vi "Main.vi"(11 "DataIn":T1) -> (3 "DataOut":T1)   [LabVIEW 2018]
doc: "Main Vi para Jogo da Velha Multiplayer - Player x Player na mesma máquina, Player x Player pela rede, Player x Computador\n[Covers: REQ05]"
uses:
  controls/Tabuleiro.ctl
  controls/DataIn.ctl
  MatchDataClasses/MatchData/MatchData.lvclass
  controls/GameOption.ctl
  controls/Table.ctl
  controls/States.ctl
  controls/LogStates.ctl
  MatchDataClasses/Local/Local.lvclass
  C:/Users/liferrei/Documents/Jogo-da-Velha/MatchDataClasses/MatchData/MatchData.lvclass
  MatchDataClasses/Remote/Remote.lvclass
  Globals.vi
panel:
  in  "Remote?":bool
  in  "Reiniciar":bool
  out "Quem joga":string
  out "Tabuleiro":T2
  # "JOGO DA VELHA"
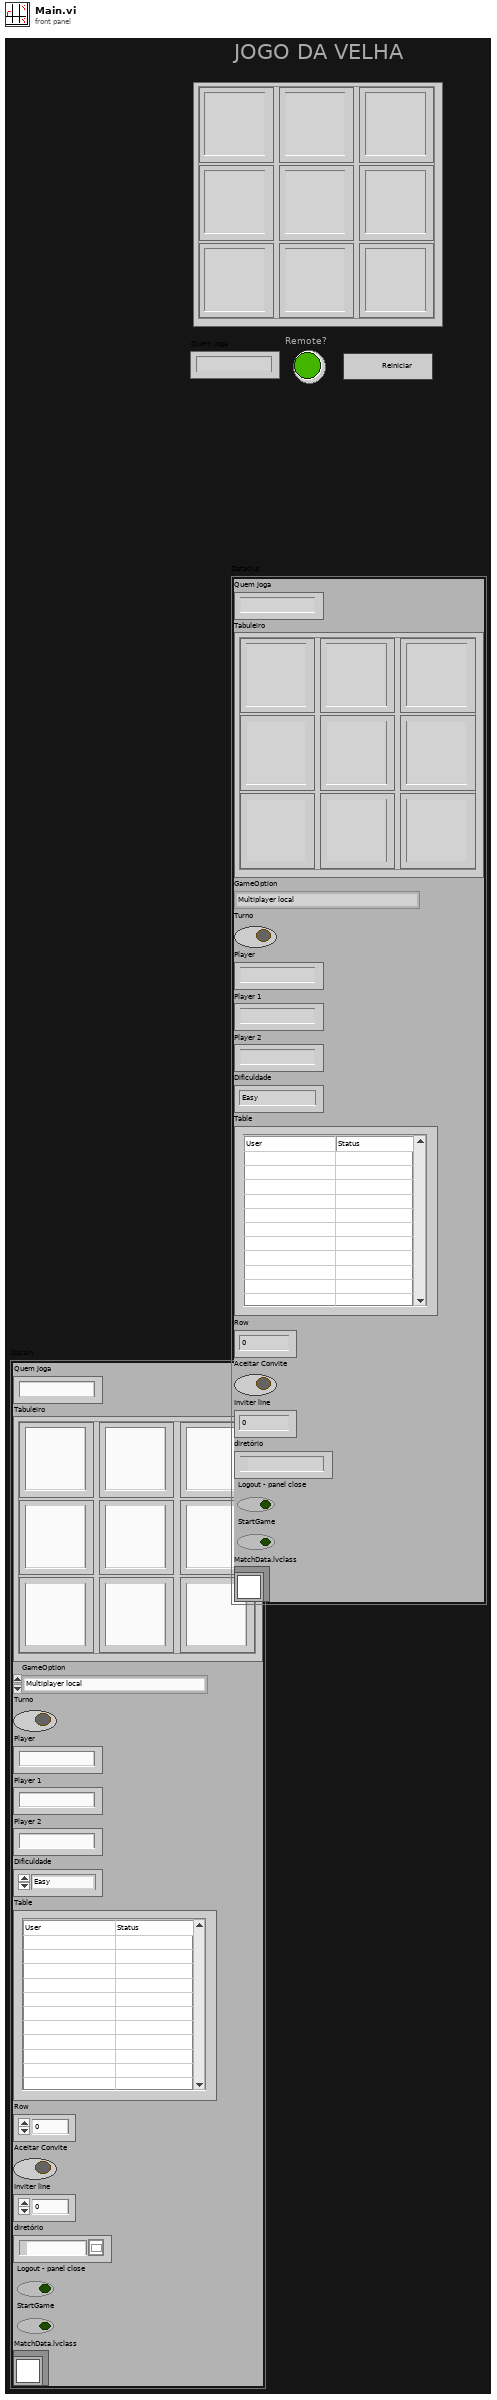
[diagram p1: front panel]
types:
  T1 = typedef "DataIn.ctl" = cluster{"Quem Joga":string, "Tabuleiro":T2, "GameOption":T3, "Turno":bool, "Player":string, "Player 1":string, "Player 2":string, "Dificuldade":enum16{"Easy", "Medium", "Hard"}, "Table":T4, "Row":u32, "Aceitar Convite":bool, "Inviter line":u32, "diretório":path, "Logout - panel close":bool, "StartGame":bool, "MatchData.lvclass":refnum<class "MatchData.lvclass">}
  T2 = typedef "Tabuleiro.ctl" = cluster{"(0,0)":string, "(1,0)":string, "(0,1)":string, "(1,1)":string, "(2,0)":string, "(1,2)":string, "(2,2)":string, "(0,2)":string, "(2,1) ":string}
  T3 = typedef "GameOption.ctl" = enum16{"Multiplayer local", "Multiplayer remoto", "Single Player", "Wait for Event", "Initialize", "Stop"}
  T4 = typedef "Table.ctl" = string[][]
  T5 = typedef "States.ctl" = enum16{"Initialize", "Player (wait for event)", "Stop", "PC", "Restart"}
  T6 = typedef "LogStates.ctl" = enum16{"Initialize", "Write", "Write (win, draw)", "Write (PC first)", "Write (Player first)", "Close"}
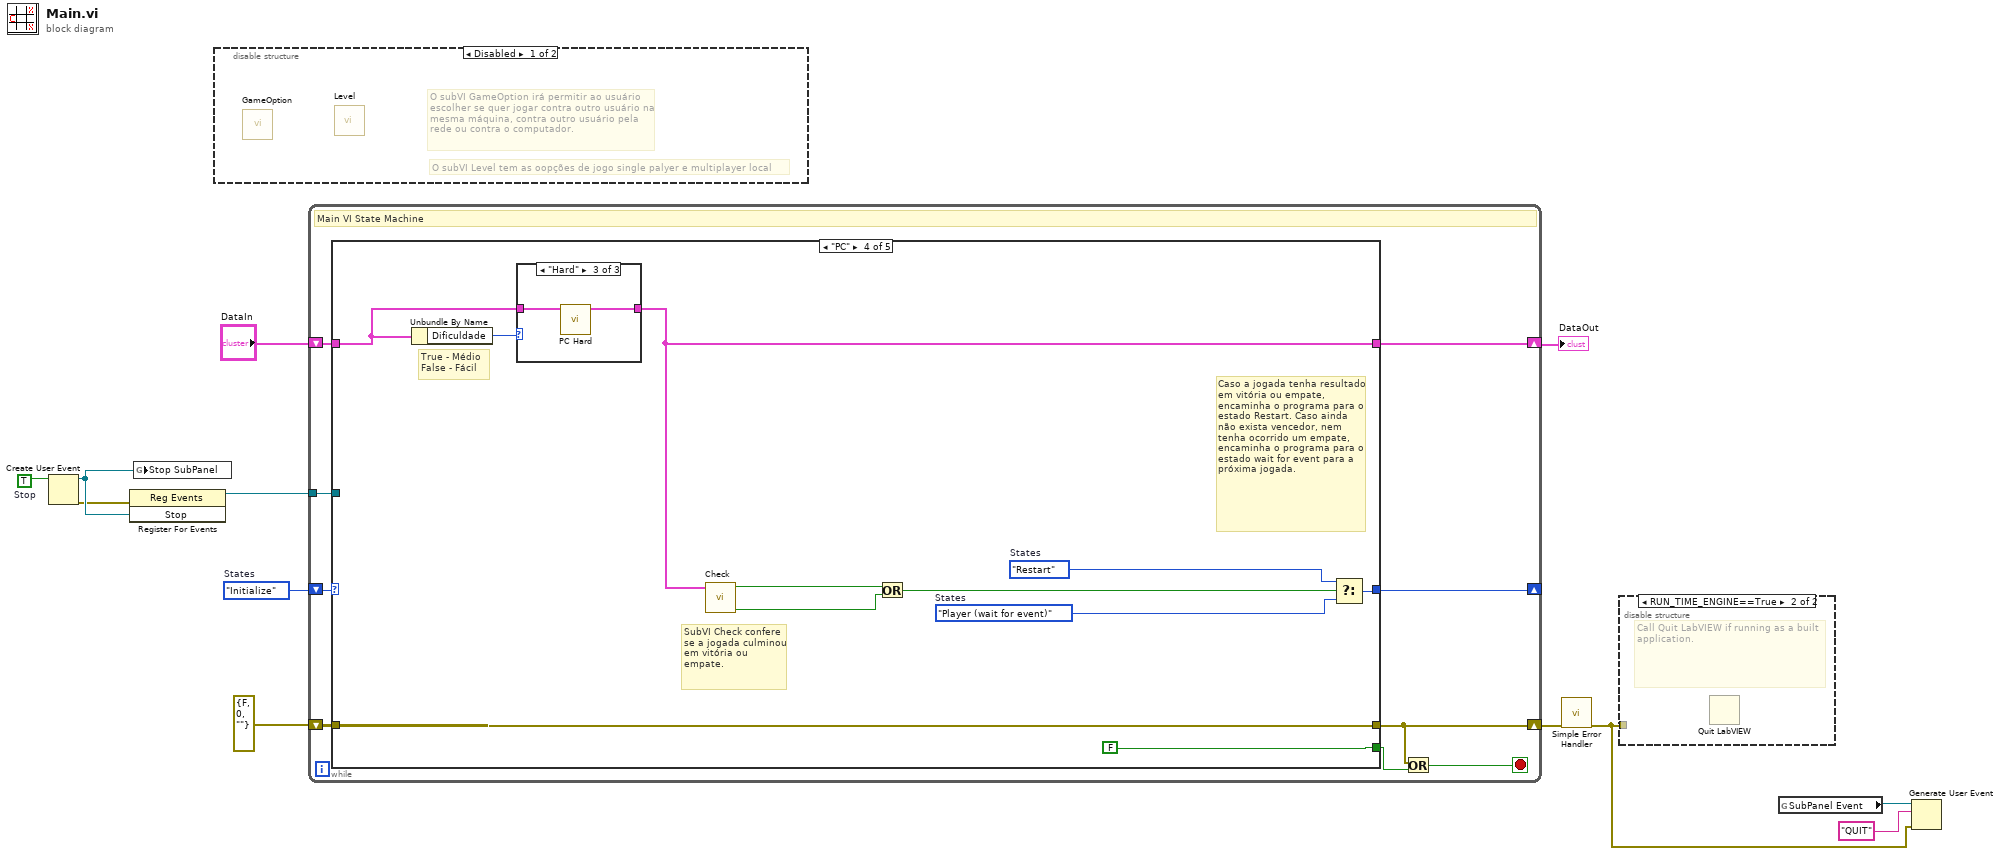
[diagram p0: block diagram]
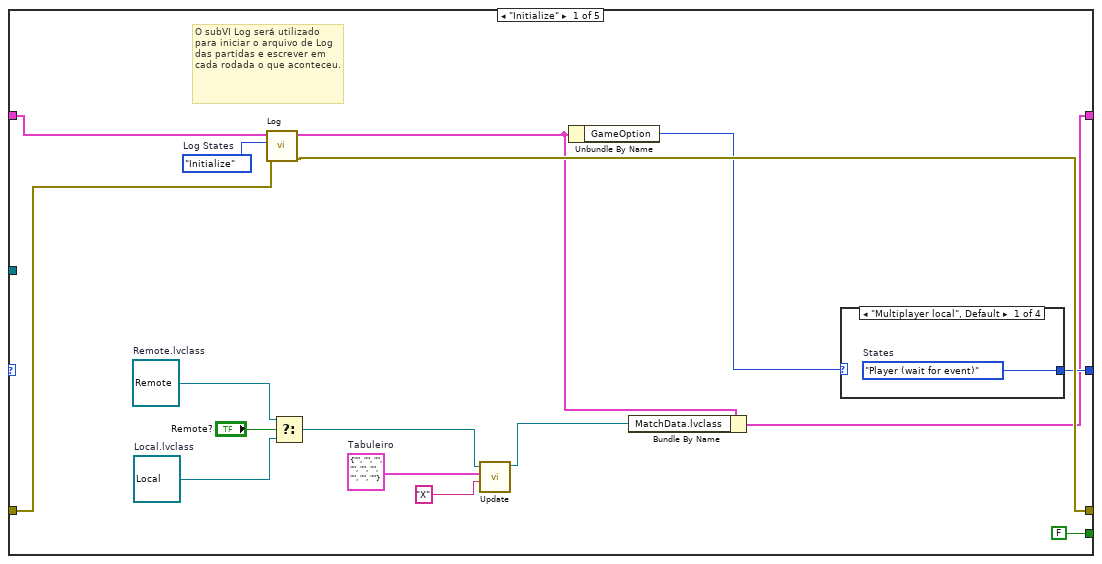
[diagram p3: hidden frame]
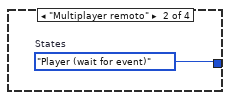
[diagram p4: hidden frame]
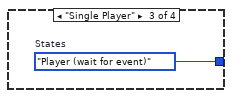
[diagram p5: hidden frame]
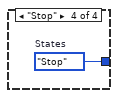
[diagram p6: hidden frame]
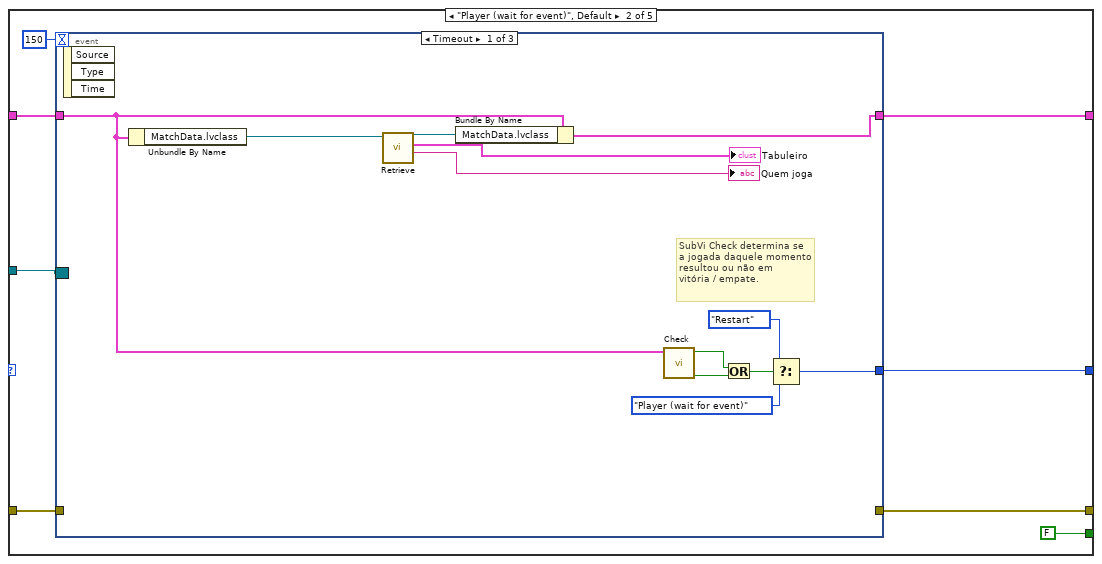
[diagram p7: hidden frame]
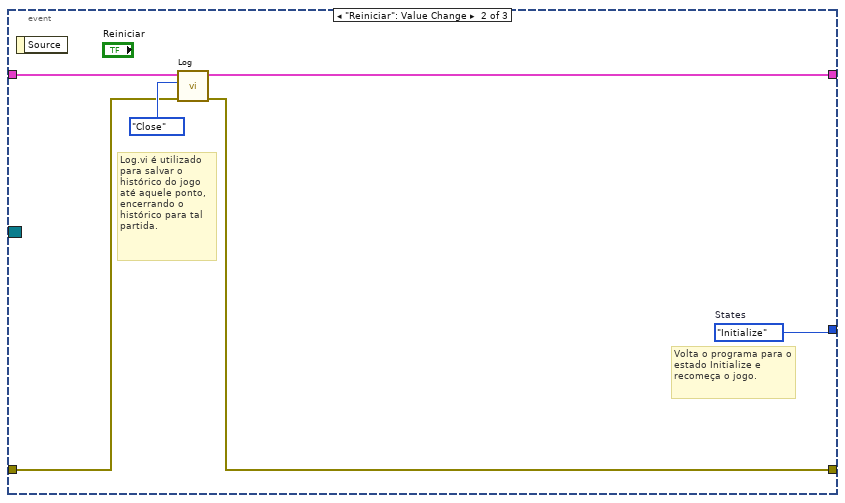
[diagram p8: hidden frame]
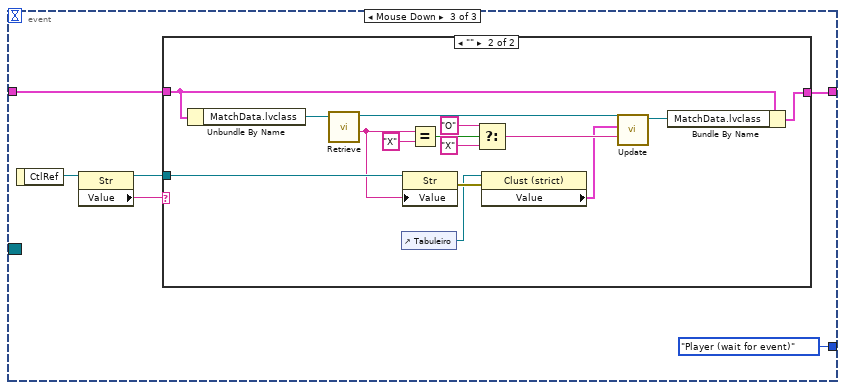
[diagram p9: hidden frame]
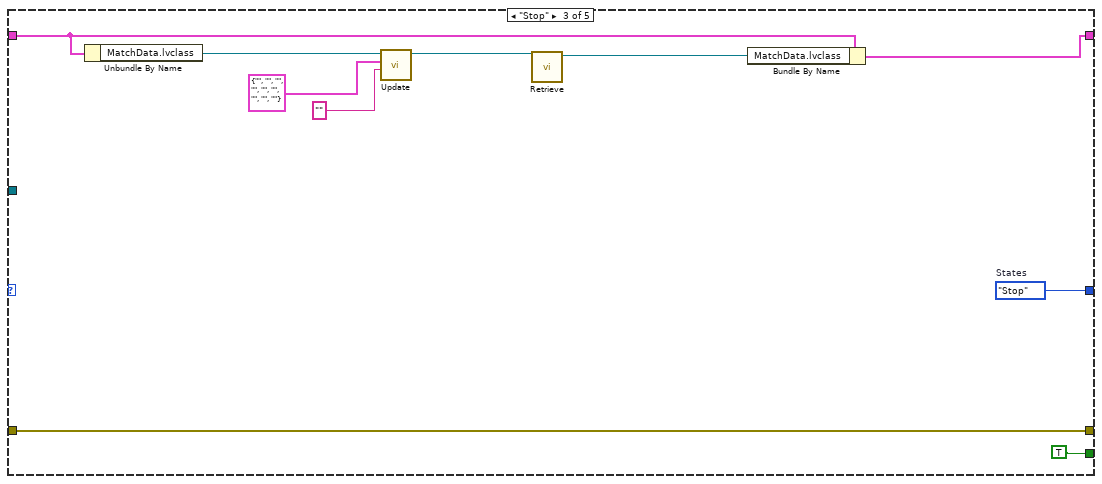
[diagram p11: hidden frame]
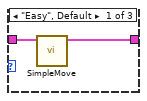
[diagram p12: hidden frame]
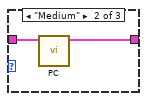
[diagram p13: hidden frame]
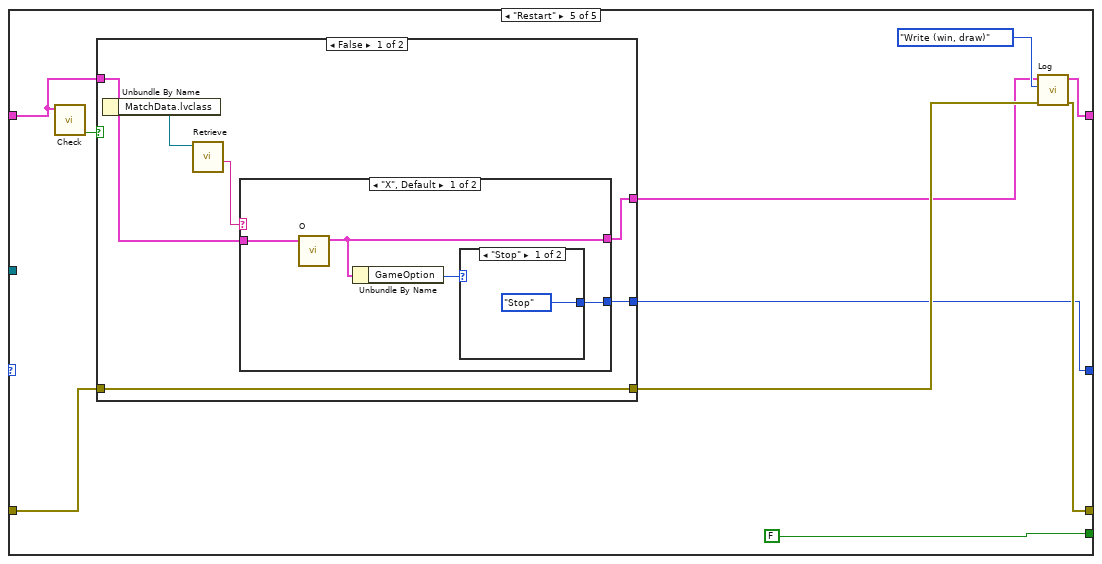
[diagram p14: hidden frame]
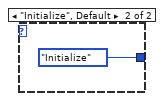
[diagram p15: hidden frame]
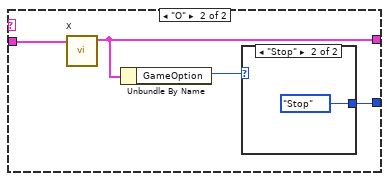
[diagram p16: hidden frame]
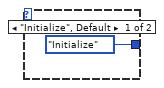
[diagram p17: hidden frame]
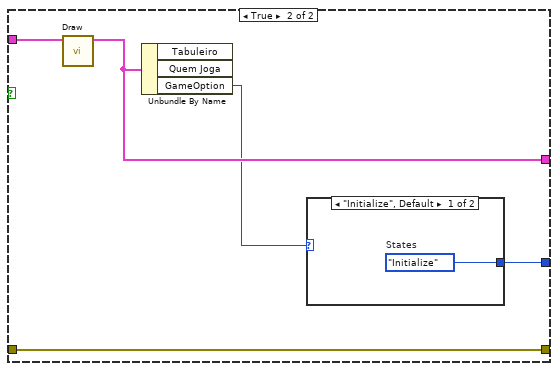
[diagram p18: hidden frame]
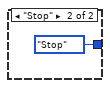
[diagram p19: hidden frame]
diagram:
  w3 = TRUE  # Stop
  w8 = States."Initialize"  # States
  n1 = Create User Event(user event datatype=w3) -> (user event=w4:refnum<user-event>, error out=w2:errorcluster)  [unwired: 1 in]
  n2 = register-events(error in=w2, w4) -> (reference out=w1:refnum<event-registration>)  [unwired: 1 in, 1 out]
  n3 = global write "Globals.vi" "Stop SubPanel"(w4) -> ()
  n4 = disable-structure shown="Disabled" {
    frame Disabled {
      # "O subVI Level tem as oopções de jogo single palyer e multiplayer local"
      # "O subVI GameOption irá permitir ao usuário escolher se quer jogar contra outro usuário na mesma máquina, contra outro usuário pela rede ou contra o computador."
      n5 = call "GameOption.vi"() -> ()  [unwired: 11 in, 1 out]
      n6 = call "Level.vi"() -> ()  [unwired: 11 in, 1 out]
    }
    frame Enabled {
    }
  }
  n7 = while {
    shift-right: [w18] -> w10
    shift-left: "DataIn" -> [w19]
    shift-right: [w16] -> w9
    shift-left: errorcluster {"status"=FALSE, "code"=0, "source"=""} ("error constant") -> [w17]
    shift-right: [w15] -> _
    shift-left: w8 -> [w20]
    tunnel: w1 -> [w13]
    stop <- w21 stop-if-true
    # "Main VI State Machine"
    n8 = case shown="\"PC\"" w20 {
      tunnel: w19 -> [w29 w48 w92 w101 w124]
      tunnel: [w22 w45 w91 w100 w119] -> w18
      tunnel: w17 -> [w37 w47 w99 w103 w123]
      tunnel: [w35 w46 w99 w103 w120] -> w16
      tunnel: [w34 w43 w98 w104 w118] -> w15
      tunnel: [FALSE FALSE TRUE FALSE FALSE] -> w14
      tunnel: w13 -> [_ w42 _ _ _]
      frame "Initialize" {
        w25 = refnum<class "Remote.lvclass"> refnum  # Remote.lvclass
        w26 = refnum<class "Local.lvclass"> refnum  # Local.lvclass
        w33 = LogStates."Initialize"  # Log States
        w32 = T2 {"(0,0)"="", "(1,0)"="", "(0,1)"="", "(1,1)"="", "(2,0)"="", "(1,2)"="", "(2,2)"="", "(0,2)"="", "(2,1) "=""}  # Tabuleiro
        # "O subVI Log será utilizado para iniciar o arquivo de Log das partidas e escrever em cada rodada o que aconteceu."
        n9 = call "Log.vi"("Error In"=w37, "Log States"=w33, "DataIn"=w29) -> ("Error Out"=w35:errorcluster, "DataOut"=w23:T1)  [unwired: 7 in]
        n10 = Select(t=w25, s="Remote?", f=w26) -> (s? t:f=w24:refnum<class "MatchData.lvclass">)
        n11 = call-dynamic "Update.vi"("Quem joga"="X" ("Quem Joga"), "Tabuleiro"=w32, "MatchData in"=w24) -> ("MatchData out"=w30:refnum<class "MatchData.lvclass">)  [unwired: 7 in, 1 out]
        n12 = Unbundle By Name(w23) -> ("GameOption"=w28:T3)
        n13 = Bundle By Name(cluster=w23, "MatchData.lvclass"=w30) -> (w22:T1)
        n14 = case shown="\"Multiplayer local\", Default" w28 {
          tunnel: [w38 w39 w40 w41] -> w34
          frame "Multiplayer local", Default {
            w38 = States."Player (wait for event)"  # States
          }
          frame "Multiplayer remoto" {
            w39 = States."Player (wait for event)"  # States
          }
          frame "Single Player" {
            w40 = States."Player (wait for event)"  # States
          }
          frame "Stop" {
            w41 = States."Stop"  # States
          }
        }
      }
      frame "Player (wait for event)", Default {
        n15 = event shown="[0] Timeout" {
          selector: w42 -> [_ _ _]
          dyn-events: _ -> [_ _ _]
          timeout: 150 -> [_ _ _]
          tunnel: w48 -> [w50 w67 w70]
          tunnel: [w57 w63 w69] -> w45
          tunnel: w47 -> [_ w65 _]
          tunnel: [_ w64 _] -> w46
          tunnel: [w51 w62 States."Player (wait for event)" ("States")] -> w43
          event Timeout {
            # "SubVi Check determina se a jogada daquele momento resultou ou não em vitória / empate."
            n16 = event-data() -> ()  [unwired: 1 in, 3 out]
            n17 = Unbundle By Name(w50) -> ("MatchData.lvclass"=w61:refnum<class "MatchData.lvclass">)
            n18 = call-dynamic "Retrieve.vi"("MatchData in"=w61) -> ("Quem joga"=→"Quem joga":string, "Tabuleiro"=→"Tabuleiro":T2, "MatchData out"=w60:refnum<class "MatchData.lvclass">)  [unwired: 7 in, 1 out]
            n19 = Bundle By Name(cluster=w50, "MatchData.lvclass"=w60) -> (w57:T1)
            n20 = call "Check.vi"("DataIn"=w50) -> ("True = Empatou"=w54:bool, "True = Ganhou"=w55:bool)  [unwired: 9 in]
            n21 = Or(x=w55, y=w54) -> (x .or. y?=w56:bool)
            n22 = Select(t=States."Restart", s=w56, f=States."Player (wait for event)") -> (s? t:f=w51:T5)
          }
          event "Reiniciar": Value Change {
            w62 = States."Initialize"  # States
            # "Log.vi é utilizado para salvar o histórico do jogo até aquele ponto, encerrando o histórico para tal partida."
            # "Volta o programa para o estado Initialize e recomeça o jogo."
            n23 = event-data() -> ()  [unwired: 1 in, 1 out]
            n24 = call "Log.vi"("Error In"=w65, "Log States"=LogStates."Close", "DataIn"=w67) -> ("Error Out"=w64:errorcluster, "DataOut"=w63:T1)  [unwired: 7 in]
          }
          event Mouse Down {
            n25 = event-data() -> ("CtlRef"=w73:refnum<vi>)  [unwired: 1 in]
            n26 = property class="Str"(reference=w73) -> (reference out=w71:refnum<vi>, "Value"=w72:string)  [unwired: 1 in, 1 out]
            n27 = case shown="\"\"" w72 {
              tunnel: w71 -> [_ w88]
              tunnel: w70 -> [w74 w77]
              tunnel: [w74 w75] -> w69
              frame "True", Default {
              }
              frame "" {
                n28 = Unbundle By Name(w77) -> ("MatchData.lvclass"=w89:refnum<class "MatchData.lvclass">)
                n29 = call-dynamic "Retrieve.vi"("MatchData in"=w89) -> ("Quem joga"=w87:string, "MatchData out"=w78:refnum<class "MatchData.lvclass">)  [unwired: 7 in, 2 out]
                n30 = control-ref of="Tabuleiro"() -> (w81:refnum<vi>)
                n31 = property class="Str"(reference=w88, "Value"=w87) -> (error out=w82:errorcluster)  [unwired: 1 in, 1 out]
                n32 = Equal?(x=w87, y="X") -> (x = y?=w85:bool)
                n33 = Select(t="O", s=w85, f="X" ("y")) -> (s? t:f=w80:string)
                n34 = property class="Clust (strict)"(reference=w81, error in=w82) -> ("Value"=w79:T2)  [unwired: 2 out]
                n35 = call-dynamic "Update.vi"("Quem joga"=w80, "Tabuleiro"=w79, "MatchData in"=w78) -> ("MatchData out"=w76:refnum<class "MatchData.lvclass">)  [unwired: 7 in, 1 out]
                n36 = Bundle By Name(cluster=w77, "MatchData.lvclass"=w76) -> (w75:T1)
              }
            }
          }
        }
      }
      frame "Stop" {
        w98 = States."Stop"  # States
        n37 = Unbundle By Name(w92) -> ("MatchData.lvclass"=w96:refnum<class "MatchData.lvclass">)
        n38 = call-dynamic "Update.vi"("Quem joga"="" ("Quem Joga"), "Tabuleiro"=T2 {"(0,0)"="", "(1,0)"="", "(0,1)"="", "(1,1)"="", "(2,0)"="", "(1,2)"="", "(2,2)"="", "(0,2)"="", "(2,1) "=""}, "MatchData in"=w96) -> ("MatchData out"=w93:refnum<class "MatchData.lvclass">)  [unwired: 7 in, 1 out]
        n39 = call-dynamic "Retrieve.vi"("MatchData in"=w93) -> ("MatchData out"=w90:refnum<class "MatchData.lvclass">)  [unwired: 7 in, 3 out]
        n40 = Bundle By Name(cluster=w92, "MatchData.lvclass"=w90) -> (w91:T1)
      }
      frame "PC" {
        w105 = States."Player (wait for event)"  # States
        w106 = States."Restart"  # States
        # "True - Médio\nFalse - Fácil"
        # "Caso a jogada tenha resultado em vitória ou empate, encaminha o programa para o estado Restart. Caso ainda não exista vencedor, nem tenha ocorrido um empate, encaminha o programa para o estado wait for event para a próxima jogada."
        # "SubVI Check confere se a jogada culminou em vitória ou empate."
        n41 = Unbundle By Name(w101) -> ("Dificuldade"=w102:enum16{"Easy", "Medium", "Hard"})
        n42 = case shown="\"Hard\"" w102 {
          tunnel: w101 -> [w111 w114 w115]
          tunnel: [w112 w113 w116] -> w100
          frame "Easy", Default {
            n43 = call "SimpleMove.vi"("DataIn"=w111) -> ("DataOut"=w112:T1)  [unwired: 10 in]
          }
          frame "Medium" {
            n44 = call "PC.vi"("DataIn"=w114) -> ("DataOut"=w113:T1)  [unwired: 10 in]
          }
          frame "Hard" {
            n45 = call "PC Hard.vi"("DataIn"=w115) -> ("DataOut"=w116:T1)  [unwired: 10 in]
          }
        }
        n46 = call "Check.vi"("DataIn"=w100) -> ("True = Empatou"=w108:bool, "True = Ganhou"=w109:bool)  [unwired: 9 in]
        n47 = Or(x=w109, y=w108) -> (x .or. y?=w107:bool)
        n48 = Select(t=w106, s=w107, f=w105) -> (s? t:f=w104:T5)
      }
      frame "Restart" {
        n49 = call "Check.vi"("DataIn"=w124) -> ("True = Empatou"=w125:bool)  [unwired: 9 in, 1 out]
        n50 = case shown="False" w125 {
          tunnel: w124 -> [w129 w149]
          tunnel: w123 -> [w132 w148]
          tunnel: [w132 w148] -> w122
          tunnel: [w131 w147] -> w117
          tunnel: [w130 w145] -> w118
          frame False {
            n51 = Unbundle By Name(w129) -> ("MatchData.lvclass"=w128:refnum<class "MatchData.lvclass">)
            n52 = call-dynamic "Retrieve.vi"("MatchData in"=w128) -> ("Quem joga"=w127:string)  [unwired: 7 in, 3 out]
            n53 = case shown="\"X\", Default" w127 {
              tunnel: w129 -> [w136 w142]
              tunnel: [w135 w141] -> w131
              tunnel: [w133 w139] -> w130
              frame "X", Default {
                n54 = call "O.vi"("DataIn"=w136) -> ("DataOut"=w135:T1)  [unwired: 10 in]
                n55 = Unbundle By Name(w135) -> ("GameOption"=w134:T3)
                n56 = case shown="\"Stop\"" w134 {
                  tunnel: [States."Stop" ("States") States."Initialize" ("States")] -> w133
                  frame "Stop" {
                  }
                  frame "Initialize", Default {
                  }
                }
              }
              frame "O" {
                n57 = call "X.vi"("DataIn"=w142) -> ("DataOut"=w141:T1)  [unwired: 10 in]
                n58 = Unbundle By Name(w141) -> ("GameOption"=w140:T3)
                n59 = case shown="\"Stop\"" w140 {
                  tunnel: [States."Initialize" ("States") States."Stop" ("States")] -> w139
                  frame "Initialize", Default {
                  }
                  frame "Stop" {
                  }
                }
              }
            }
          }
          frame True {
            n60 = call "Draw.vi"("DataIn"=w149) -> ("DataOut"=w147:T1)  [unwired: 10 in]
            n61 = Unbundle By Name(w147) -> ("GameOption"=w146:T3)  [unwired: 2 out]
            n62 = case shown="\"Initialize\", Default" w146 {
              tunnel: [w150 States."Stop" ("States")] -> w145
              frame "Initialize", Default {
                w150 = States."Initialize"  # States
              }
              frame "Stop" {
              }
            }
          }
        }
        n63 = call "Log.vi"("Error In"=w122, "Log States"=LogStates."Write (win, draw)", "DataIn"=w117) -> ("Error Out"=w120:errorcluster, "DataOut"=w119:T1)  [unwired: 7 in]
      }
    }
    n64 = Or(x=w16, y=w14) -> (x .or. y?=w21:bool)
  }
  "DataOut" <- w10
  n65 = call <vilib>:"Simple Error Handler.vi"("error in (no error)"=w9) -> ("error out"=w5:errorcluster)  [unwired: 4 in, 4 out]
  n66 = disable-structure shown="RUN_TIME_ENGINE==True" {
    disable-tunnel: w5 -> [_ _]
    frame condition #0 (active) {
    }
    frame condition #1 {
      # "Call Quit LabVIEW if running as a built application."
      n67 = Quit LabVIEW() -> ()  [unwired: 1 in]
    }
  }
  n68 = global read "Globals.vi" "SubPanel Event"() -> (w7:refnum<user-event>)
  n69 = Generate User Event(user event=w7, event data cluster="QUIT" ("event data"), error in=w5) -> ()  [unwired: 1 in, 2 out]
